vi "BT Rx Test Fetch Results.vi"(8 "error in (no error)":errorcluster, 11 "niDTS BT Rx Test in":refnum<class "niDTS BT Rx Test.lvclass">) -> (0 "error out":errorcluster, 2 "Results":T1, 3 "niDTS BT Rx Test out":refnum<class "niDTS BT Rx Test.lvclass">)   [LabVIEW 2015, in "niDTS BT.lvlib" / "niDTS BT Rx Test.lvclass"]
uses:
  niDTS BT Rx Test.lvclass
  Includes/niDTS BT Rx Test INC Results.ctl
  niDTS BT Rx Test.lvclass/niDTS BT Rx Test.ctl
  niDTS BT.lvlib
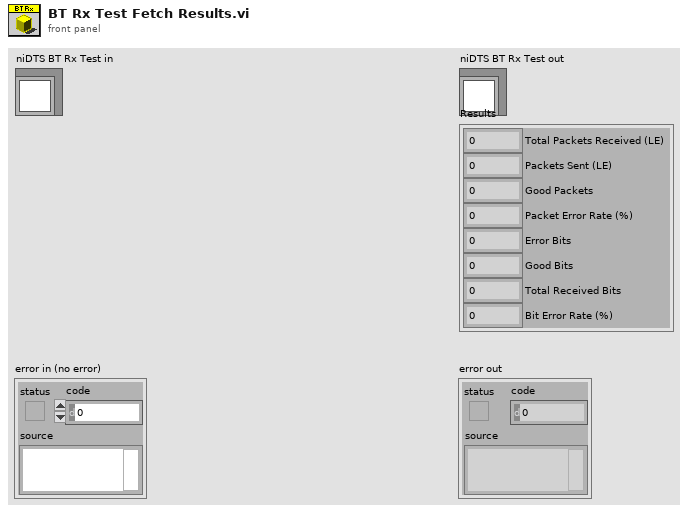
[diagram p1: front panel]
types:
  T1 = typedef "niDTS BT.lvlib/niDTS BT Rx Test INC Results.ctl" = cluster{"Total Packets Received (LE)":i32, "Packets Sent (LE)":dbl, "Good Packets":dbl, "Packet Error Rate (%)":dbl, "Error Bits":u32, "Good Bits":u32, "Total Received Bits":u32, "Bit Error Rate (%)":dbl}
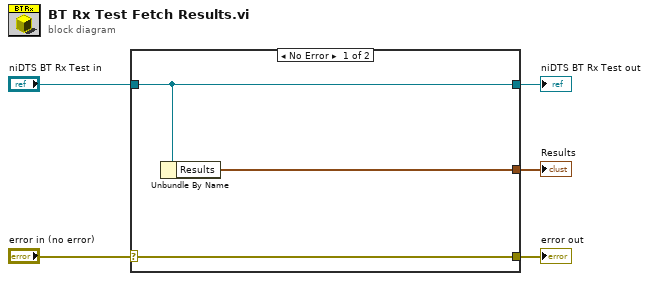
[diagram p0: block diagram]
diagram:
  n1 = case shown="No Error" "error in (no error)" {
    selector: "error in (no error)" -> [w8 w9]
    tunnel: [w8 w9] -> w4
    tunnel: [w7 w10] -> w2
    tunnel: "niDTS BT Rx Test in" -> [w7 w10]
    tunnel: [w6 _] -> w1
    frame No Error {
      n2 = Unbundle By Name(w7) -> ("Results"=w6:T1)
    }
    frame Error {
    }
  }
  "error out" <- w4
  "niDTS BT Rx Test out" <- w2
  "Results" <- w1
